vi "DtCreateAoutChan.vi"(2 "Range Min":dbl=-10.0, 3 "Range Max":dbl=10.0, 5 "Board Name":string, 7 "Channel":string="Ain 0", 9 "Element":u32, 11 "error in (no error)":errorcluster) -> (4 "Task out":i32, 8 "Actual Number of Channels":u32, 15 "error out":errorcluster)   [LabVIEW 2022 SP3]
doc: "Creates one or more virtual analog output channels to output voltage. If your device supports streaming digital data through the analog output subsystem, use the Analog Output - Raw instance of this VI."
uses:
  DtLvLink.lvlib
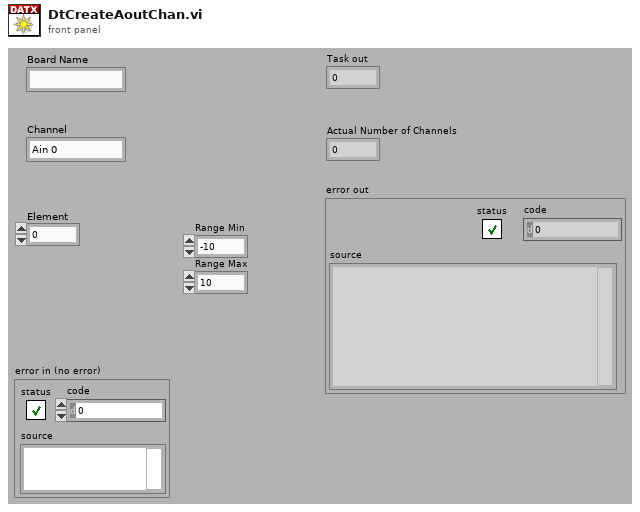
[diagram p1: front panel]
types:
  T1 = enum32{"AnalogInput", "AnalogOutput", "DigitalInput", "DigitalOutput", "Quadrature", "CounterTimer"}
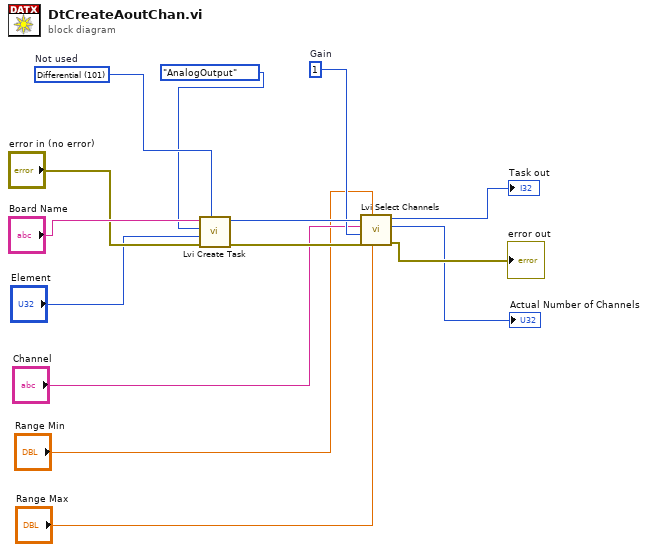
[diagram p0: block diagram]
diagram:
  w3 = 101 items=["SingleEnded"=100, "Differential"=101]  # Not used
  w12 = u32 1  # Gain
  n1 = call "Lvi Create Task.vi"("SEorDiff"=w3, "error in (no error)"="error in (no error)", "SubSysIndex"="Element", "ChanType"=T1."AnalogOutput", "BoardName"="Board Name") -> ("error out"=w13:errorcluster, "TaskRef"=w14:i32)  [unwired: 4 in, 1 out]
  n2 = call "Lvi Select Channels.vi"("MaxRange"="Range Max", "MinRange"="Range Min", "error in (no error)"=w13, "Gain"=w12, "ChanListStr"="Channel", "TaskRef"=w14) -> ("error out"=→"error out":errorcluster, "ActualNumChannels"=→"Actual Number of Channels":u32, "TaskRef out"=→"Task out":i32)  [unwired: 2 in, 1 out]
